vi "forceplate_V1.vi"() -> ()   [LabVIEW 2014]
uses:
  typedef.ctl
  <vilib>/Utility/error.llb/DialogType.ctl
  <vilib>/DAQmx/read.llb/DAQmx Read (Analog 1D DBL NChan 1Samp).vi
  <vilib>/DAQmx/create/channels.llb/DAQmx Create Channel (AI-Voltage-Basic).vi
  <vilib>/DAQmx/miscellaneous.llb/DAQmx Fill In Error Info.vi
  <vilib>/Utility/file.llb/Write To Spreadsheet File (DBL).vi
  <vilib>/DAQmx/configure/timing.llb/DAQmx Timing (Sample Clock).vi
panel:
  in  "save":bool
  out "Kilogram (kg)":dbl
  out "Peak force (N) landing phase":dbl
  out "Peak force (N) contact phase":dbl
  out "Flight time (s)":dbl
  out "Jump height (m)":dbl
  in  "Jump#":dbl=1.0
  out "sampling rate for last data":dbl=1000.0
  out "average":dbl
  out "Slide":dbl(slide) scale=0.0..3000.0
  in  "start":bool
  in  "calibrate":bool
  out "scale":dbl
  out "known":dbl
  out "zero":dbl
  in  "Calibration\n weight (kg)":dbl
  out "Newton (N)":dbl
  in  "Stop":bool
  out "Waveform Graph":dbl[](graph)
  in  "Sample rate":dbl=1000.0
  in  "Sample Clock Source":tag="OnboardClock"
  in  "Terminal Configuration":i32(ring)=-1 items=["default"=-1, "RSE"=10083, "NRSE"=10078, "Differential"=10106, "Pseudodifferential"=12529]
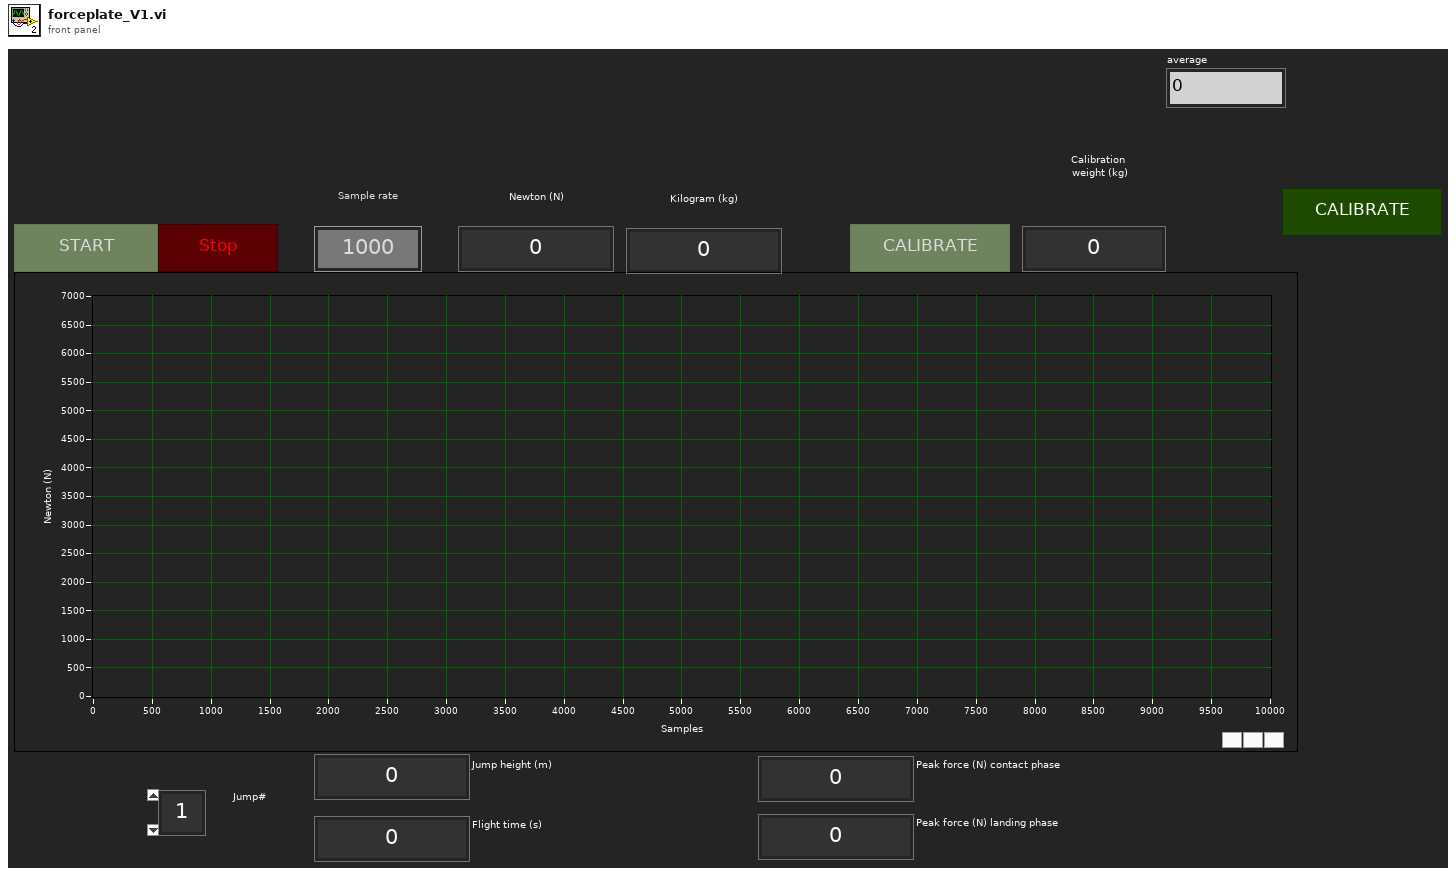
[diagram p1: front panel]
types:
  T1 = typedef "typedef.ctl" = enum16{"display", "read", "calibrate", "wait", "Init"}
  T2 = enum8{"Enabled", "Disabled", "Disabled and Grayed Out"}
  T3 = typedef "DialogType.ctl" = u16
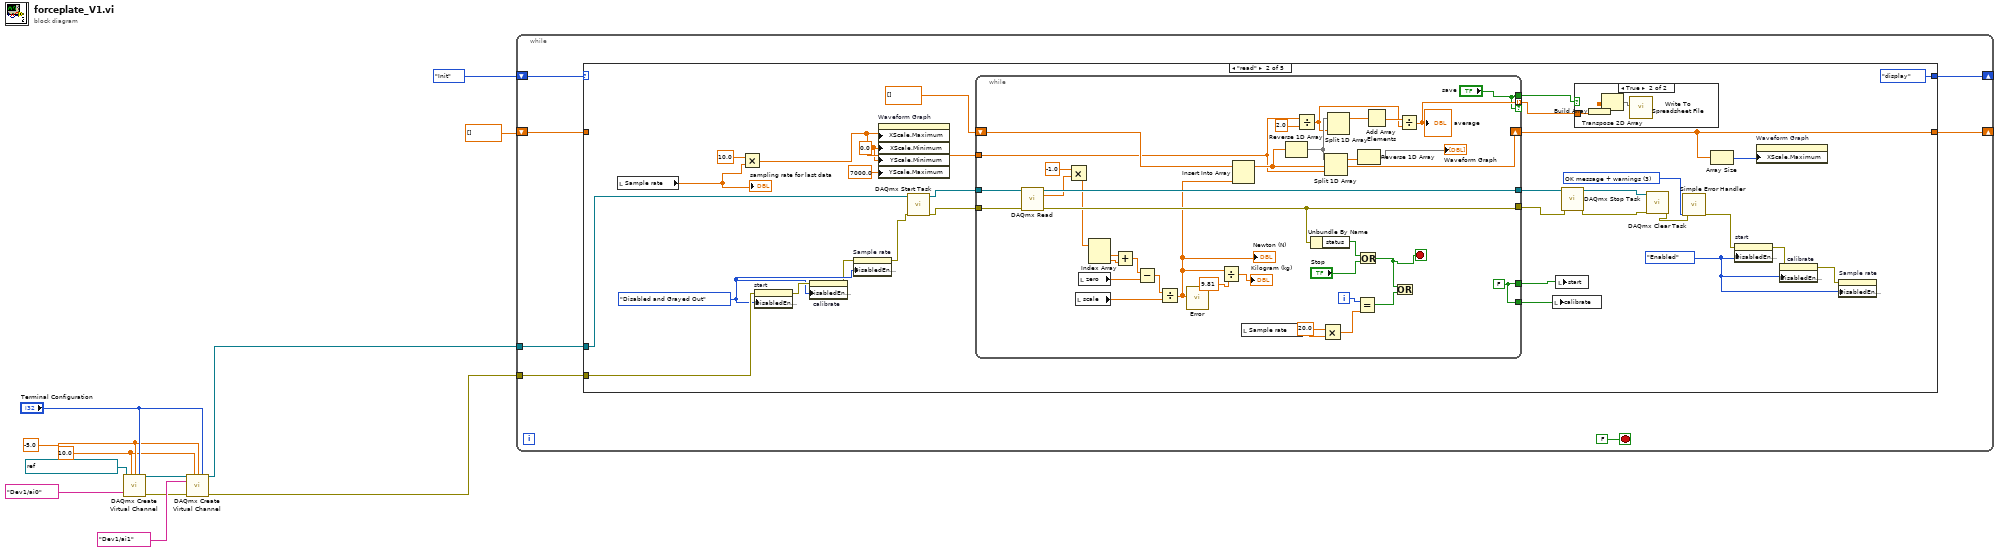
[diagram p0: block diagram]
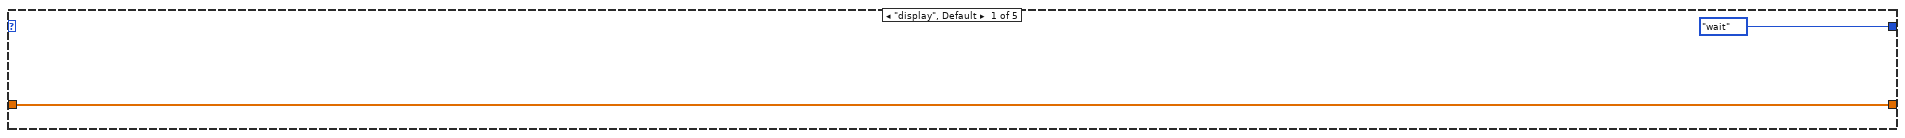
[diagram p2: hidden frame]
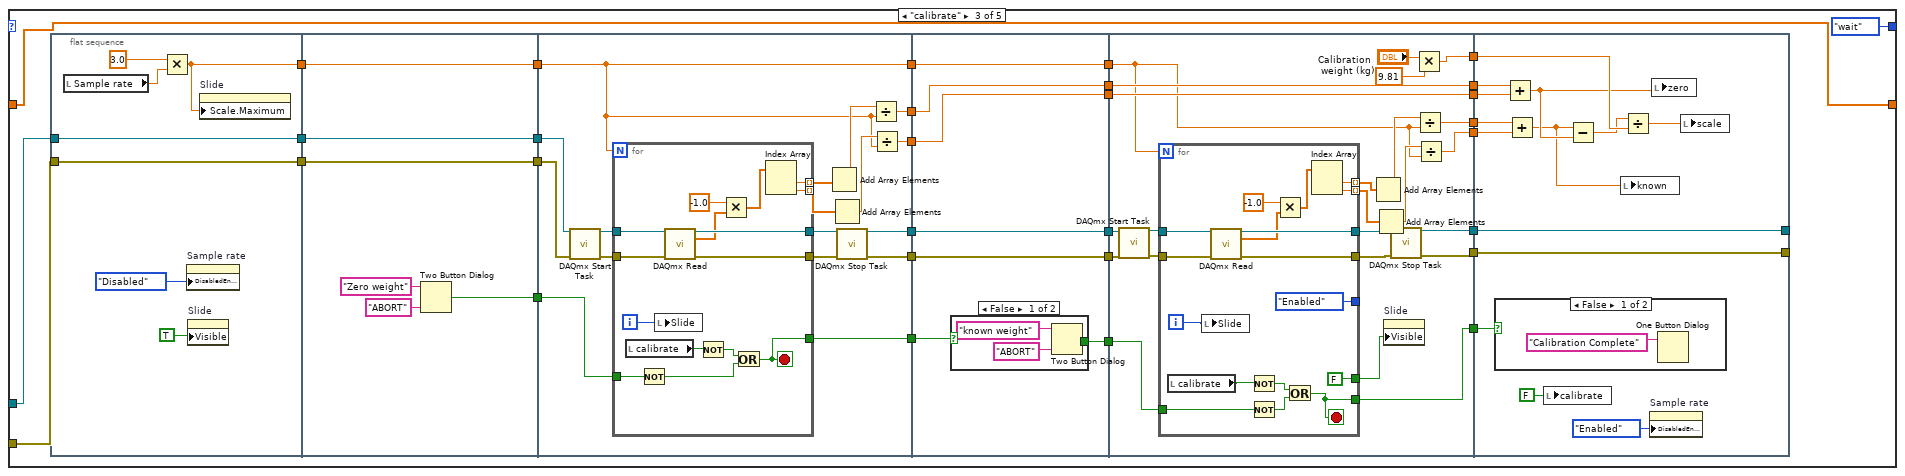
[diagram p4: hidden frame]
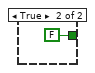
[diagram p5: hidden frame]
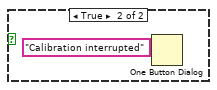
[diagram p6: hidden frame]
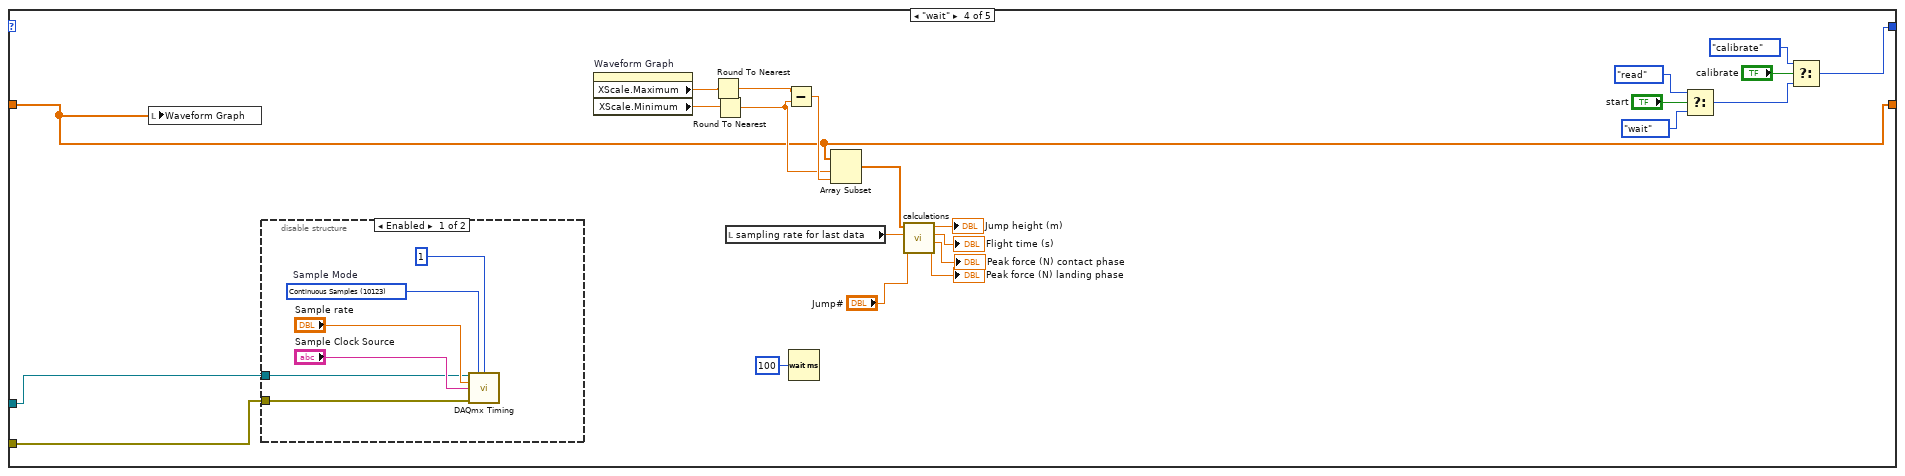
[diagram p7: hidden frame]
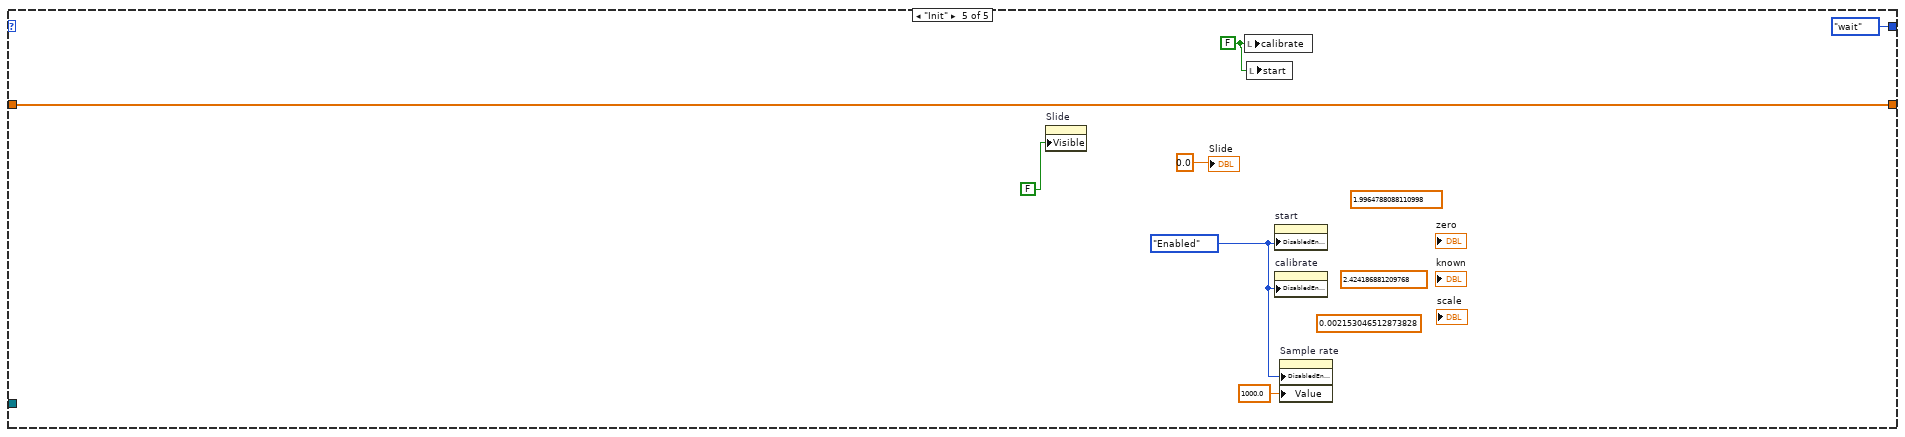
[diagram p9: hidden frame]
diagram:
  w6 = -5.0 ("Min Voltage")
  w5 = 10.0 ("Max Voltage")
  n1 = call-poly <vilib>:"DAQmx Create Virtual Channel.vi"("task in"=refnum<k21> "ProjectVoltageTask", "maximum value"=w5, "minimum value"=w6, "input terminal configuration"="Terminal Configuration", "physical channels"=tag "Dev1/ai0" ("Physical Channel")) -> ("task out"=w9:refnum<k21>, "error out"=w8:errorcluster)  [unwired: 9 in]
  n2 = call-poly <vilib>:"DAQmx Create Virtual Channel.vi"("task in"=w9, "maximum value"=w5, "minimum value"=w6, "input terminal configuration"="Terminal Configuration", "physical channels"=tag "Dev1/ai1" ("Physical Channel 2"), "error in"=w8) -> ("task out"=w2:refnum<k21>, "error out"=w1:errorcluster)  [unwired: 8 in]
  n3 = while {
    shift-right: [w18] -> _
    shift-left: typedef."Init" ("Enum") -> [w19]
    tunnel: w2 -> [w17]
    tunnel: w1 -> [w16]
    shift-right: [w15] -> _
    shift-left: dbl[] [] -> [w14]
    stop <- FALSE stop-if-true
    n4 = case shown="\"read\"" w19 {
      tunnel: [typedef."wait" ("Enum") typedef."display" ("Enum") typedef."wait" ("Enum") w253 typedef."wait" ("Enum")] -> w18
      tunnel: w17 -> [_ w43 w100 w251 _]
      tunnel: w16 -> [_ w37 w99 w250 _]
      tunnel: [w20 w24 w97 w243 w270] -> w15
      tunnel: w14 -> [w20 _ w97 w243 w270]
      frame "display", Default {
      }
      frame "read" {
        w28 = T2."Enabled" ("Disabled")
        w32 = T2."Disabled and Grayed Out" ("Disabled")
        w27 = 0.0 ("Y Scale.Range:Minimum")
        w49 = T3 3 items=["no dialog", "OK message", "continue or stop message", "OK message + warnings", "continue/stop + warnings"] ("type of dialog (OK msg:1)")
        n5 = local read "Sample rate"() -> (w33:dbl)
        "sampling rate for last data" <- w33
        n6 = Multiply(x=10.0, y=w33) -> (x*y=w40:dbl)
        n7 = property on="start" class="Bool (strict)"(error in=w37, "DisabledEnum"=w32) -> (error out=w35:errorcluster)  [unwired: 1 in, 1 out]
        n8 = property on="calibrate" class="Bool (strict)"(error in=w35, "DisabledEnum"=w32) -> (error out=w30:errorcluster)  [unwired: 1 in, 1 out]
        n9 = property on="Sample rate" class="DigNum (strict)"(error in=w30, "DisabledEnum"=w32) -> (error out=w31:errorcluster)  [unwired: 1 in, 1 out]
        n10 = property on="Waveform Graph" class="WFGraph (strict)"("XScale.Maximum"=w40, "XScale.Minimum"=w27, "YScale.Minimum"=w27, "YScale.Maximum"=7000.0 ("Y Scale.Range:Maximum")) -> ()  [unwired: 2 in, 2 out]
        n11 = call <vilib>:"DAQmx Start Task.vi"("task/channels in"=w43, "error in"=w31) -> ("task out"=w51:refnum<k21>, "error out"=w52:errorcluster)  [unwired: 12 in]
        n12 = while {
          tunnel: w51 -> [w92]
          tunnel: w52 -> [w91]
          tunnel: [w90] -> w45
          tunnel: [w88] -> w46
          shift-right: [w72] -> w24
          shift-left: dbl[] [] -> [w86]
          tunnel: w40 -> [w65]
          tunnel: [w67] -> w39
          tunnel: [w67] -> w38
          tunnel: [w57] -> w22 mode=indexing if="save"
          tunnel: ["save"] -> w23
          i -> [w76]
          stop <- w68 stop-if-true
          w67 = FALSE ("start")
          n13 = call-poly <vilib>:"DAQmx Read.vi"("task/channels in"=w92, "error in"=w91) -> ("task out"=w90:refnum<k21>, "data"=w83:dbl[], "error out"=w88:errorcluster)  [unwired: 11 in]
          n14 = Multiply(x=-1.0, y=w83) -> (x*y=w82:dbl[])
          n15 = local read "scale"() -> (w79:dbl)
          n16 = local read "zero"() -> (w81:dbl)
          n17 = Index Array(array=w82) -> (element #1=w77:dbl, element #2=w78:dbl)  [unwired: 2 in]
          n18 = Add(x=w77, y=w78) -> (x+y=w69:dbl)
          n19 = Subtract(x=w69, y=w81) -> (x-y=w80:dbl)
          n20 = Divide(x=w80, y=w79) -> (x/y=w58:dbl)
          "Newton (N)" <- w58
          n21 = call "Error.vi"("Newton (N)"=w58) -> ()  [unwired: 10 in, 1 out]
          n22 = Divide(x=w58, y=9.81) -> (x/y=→"Kilogram (kg)":dbl)
          n23 = Insert Into Array(array=w86, new element=w58) -> (w72:dbl[])  [unwired: 1 in]
          n24 = local read "Sample rate"() -> (w75:dbl)
          n25 = Reverse 1D Array(array=w72) -> (reversed array=w66:dbl[])
          n26 = Divide(x=w65, y=2.0) -> (x/y=w61:dbl)
          n27 = Unbundle By Name(w88) -> ("status"=w87:bool)
          n28 = Multiply(x=20.0, y=w75) -> (x*y=w73:dbl)
          n29 = Split 1D Array(array=w66, index=w65) -> (first subarray=w85:dbl[])  [unwired: 1 out]
          n30 = Split 1D Array(array=w66, index=w61) -> (first subarray=w63:dbl[])  [unwired: 1 out]
          n31 = Equal?(x=w76, y=w73) -> (x = y?=w70:bool)
          n32 = Or(x=w87, y="Stop") -> (x .or. y?=w68:bool)
          n33 = Reverse 1D Array(array=w85) -> (reversed array=→"Waveform Graph":dbl[])
          n34 = Add Array Elements(numeric array=w63) -> (sum=w62:dbl)
          n35 = Or(x=w68, y=w70) -> ()  [unwired: 1 out]
          n36 = Divide(x=w62, y=w61) -> (x/y=w57:dbl)
          "average" <- w57
        }
        n37 = local write "calibrate"(w38) -> ()
        n38 = local write "start"(w39) -> ()
        n39 = call <vilib>:"DAQmx Stop Task.vi"("task/channels in"=w45, "error in"=w46) -> ("task out"=w48:refnum<k21>, "error out"=w47:errorcluster)  [unwired: 12 in]
        n40 = case shown="True" w23 {
          tunnel: w22 -> [_ w55]
          frame False {
          }
          frame True {
            n41 = Build Array(w55) -> (w54:dbl[][])
            n42 = Transpose 2D Array(2D array=w54) -> (transposed array=w53:dbl[][])
            n43 = call-poly <vilib>:"Write To Spreadsheet File.vi"("2D data"=w53) -> ()  [unwired: 7 in, 1 out]
          }
        }
        n44 = call <vilib>:"DAQmx Clear Task.vi"("task in"=w48, "error in"=w47) -> ("error out"=w44:errorcluster)  [unwired: 13 in]
        n45 = call <vilib>:"Simple Error Handler.vi"("type of dialog (OK msg:1)"=w49, "error in (no error)"=w44) -> ("error out"=w36:errorcluster)  [unwired: 3 in, 4 out]
        n46 = Array Size(array=w24) -> (size(s)=w25:i32)
        n47 = property on="start" class="Bool (strict)"(error in=w36, "DisabledEnum"=w28) -> (error out=w34:errorcluster)  [unwired: 1 in, 1 out]
        n48 = property on="Waveform Graph" class="WFGraph (strict)"("XScale.Maximum"=w25) -> ()  [unwired: 2 in, 2 out]
        n49 = property on="calibrate" class="Bool (strict)"(error in=w34, "DisabledEnum"=w28) -> (error out=w29:errorcluster)  [unwired: 1 in, 1 out]
        n50 = property on="Sample rate" class="DigNum (strict)"(error in=w29, "DisabledEnum"=w28) -> ()  [unwired: 1 in, 2 out]
      }
      frame "calibrate" {
        n51 = flat-sequence {
          tunnel: w99 -> [w129]
          tunnel: w100 -> [w130]
          tunnel: [w130] -> w123
          tunnel: [w129] -> w122
          tunnel: [w124] -> w121
          tunnel: [w136] -> w120
          tunnel: [w135] -> w119
          tunnel: w123 -> [w136]
          tunnel: w122 -> [w135]
          tunnel: [w131] -> w118
          tunnel: w121 -> [w131]
          tunnel: [w132] -> w95
          tunnel: w120 -> [w141]
          tunnel: w119 -> [w140]
          tunnel: [w149] -> w117
          tunnel: [w148] -> w116
          tunnel: [w146] -> w115
          tunnel: [w144] -> w114
          tunnel: [w139] -> w113
          tunnel: w118 -> [w139]
          tunnel: w95 -> [w138]
          tunnel: [w137] -> w94
          tunnel: w117 -> [w172]
          tunnel: w116 -> [w171]
          tunnel: [w175] -> w112
          tunnel: w115 -> [w175]
          tunnel: [w174] -> w111
          tunnel: w114 -> [w174]
          tunnel: [w173] -> w110
          tunnel: w113 -> [w173]
          tunnel: [w172] -> w109
          tunnel: [w171] -> w108
          tunnel: w94 -> [w170]
          tunnel: [w169] -> w93
          tunnel: w112 -> [w194]
          tunnel: w111 -> [w192]
          tunnel: w110 -> [w183]
          tunnel: w109 -> [w196]
          tunnel: w108 -> [w195]
          tunnel: [w198] -> w107
          tunnel: [w197] -> w106
          tunnel: [w185] -> w105
          tunnel: [w196] -> w104
          tunnel: [w195] -> w103
          tunnel: [w188] -> w102
          tunnel: [w187] -> w101
          tunnel: [w182] -> w96
          tunnel: w93 -> [w180]
          tunnel: w107 -> [w229]
          tunnel: w106 -> [w228]
          tunnel: w105 -> [w233]
          tunnel: w104 -> [w231]
          tunnel: w103 -> [w230]
          tunnel: w102 -> [w223]
          tunnel: w101 -> [w232]
          tunnel: [w223] -> _
          tunnel: [w232] -> _
          tunnel: w96 -> [w220]
          frame #0 {
            n52 = local read "Sample rate"() -> (w127:dbl)
            n53 = Multiply(x=3.0, y=w127) -> (x*y=w124:dbl)
            n54 = property on="Sample rate" class="DigNum (strict)"("DisabledEnum"=T2."Disabled" ("Disabled")) -> ()  [unwired: 2 in, 2 out]
            n55 = property on="Slide" class="Slide (strict)"("Visible"=TRUE) -> ()  [unwired: 2 in, 2 out]
            n56 = property on="Slide" class="Slide (strict)"("Scale.Maximum"=w124) -> ()  [unwired: 2 in, 2 out]
          }
          frame #1 {
            n57 = Two Button Dialog(message="Zero weight", 1:"ABORT" ("F button name (\"Cancel\")")) -> (T button?=w132:bool)  [unwired: 1 in]
          }
          frame #2 {
            n58 = call <vilib>:"DAQmx Start Task.vi"("task/channels in"=w141, "error in"=w140) -> ("task out"=w142:refnum<k21>, "error out"=w143:errorcluster)  [unwired: 12 in]
            n59 = for {
              N: w139 -> [_]
              tunnel: w142 -> [w167]
              tunnel: w143 -> [w166]
              tunnel: [w162] -> w153 mode=indexing
              tunnel: [w165] -> w152 mode=indexing
              tunnel: [w164] -> w147
              tunnel: [w163] -> w145
              tunnel: w138 -> [w158]
              tunnel: [w156] -> w137
              i -> [w159]
              stop <- w156 stop-if-true
              n60 = local read "calibrate"() -> (w157:bool)
              n61 = Not(x=w158) -> (.not. x?=w155:bool)
              n62 = local write "Slide"(w159) -> ()
              n63 = call-poly <vilib>:"DAQmx Read.vi"("task/channels in"=w167, "error in"=w166) -> ("task out"=w164:refnum<k21>, "data"=w161:dbl[], "error out"=w163:errorcluster)  [unwired: 11 in]
              n64 = Not(x=w157) -> (.not. x?=w154:bool)
              n65 = Multiply(x=-1.0, y=w161) -> (x*y=w160:dbl[])
              n66 = Or(x=w154, y=w155) -> (x .or. y?=w156:bool)
              n67 = Index Array(array=w160) -> (element #1=w162:dbl, element #2=w165:dbl)  [unwired: 2 in]
            }
            n68 = Add Array Elements(numeric array=w153) -> (sum=w151:dbl)
            n69 = Add Array Elements(numeric array=w152) -> (sum=w150:dbl)
            n70 = call <vilib>:"DAQmx Stop Task.vi"("task/channels in"=w147, "error in"=w145) -> ("task out"=w146:refnum<k21>, "error out"=w144:errorcluster)  [unwired: 12 in]
            n71 = Divide(x=w151, y=w139) -> (x/y=w149:dbl)
            n72 = Divide(x=w150, y=w139) -> (x/y=w148:dbl)
          }
          frame #3 {
            n73 = case shown="False" w170 {
              tunnel: [w176 FALSE ("T button?")] -> w169
              frame False {
                n74 = Two Button Dialog(message="known weight", 1:"ABORT" ("F button name (\"Cancel\")")) -> (T button?=w176:bool)  [unwired: 1 in]
              }
              frame True {
              }
            }
          }
          frame #4 {
            n75 = call <vilib>:"DAQmx Start Task.vi"("task/channels in"=w194, "error in"=w192) -> ("task out"=w193:refnum<k21>, "error out"=w191:errorcluster)  [unwired: 12 in]
            n76 = for {
              N: w183 -> [_]
              tunnel: w193 -> [w218]
              tunnel: w191 -> [w217]
              tunnel: [w216] -> w200 mode=indexing
              tunnel: [w215] -> w199 mode=indexing
              tunnel: [T2."Enabled" ("Disabled")] -> _
              tunnel: [w213] -> w190
              tunnel: [w212] -> w189
              tunnel: [w203] -> w182
              tunnel: [FALSE ("Visible")] -> w181
              tunnel: w180 -> [w204]
              i -> [w209]
              stop <- w203 stop-if-true
              n77 = local read "calibrate"() -> (w207:bool)
              n78 = local write "Slide"(w209) -> ()
              n79 = call-poly <vilib>:"DAQmx Read.vi"("task/channels in"=w218, "error in"=w217) -> ("task out"=w213:refnum<k21>, "data"=w211:dbl[], "error out"=w212:errorcluster)  [unwired: 11 in]
              n80 = Not(x=w207) -> (.not. x?=w205:bool)
              n81 = Not(x=w204) -> (.not. x?=w206:bool)
              n82 = Multiply(x=-1.0, y=w211) -> (x*y=w210:dbl[])
              n83 = Or(x=w205, y=w206) -> (x .or. y?=w203:bool)
              n84 = Index Array(array=w210) -> (element #1=w216:dbl, element #2=w215:dbl)  [unwired: 2 in]
            }
            n85 = Add Array Elements(numeric array=w200) -> (sum=w201:dbl)
            n86 = Add Array Elements(numeric array=w199) -> (sum=w202:dbl)
            n87 = property on="Slide" class="Slide (strict)"("Visible"=w181) -> ()  [unwired: 2 in, 2 out]
            n88 = call <vilib>:"DAQmx Stop Task.vi"("task/channels in"=w190, "error in"=w189) -> ("task out"=w188:refnum<k21>, "error out"=w187:errorcluster)  [unwired: 12 in]
            n89 = Multiply(x="Calibration\n weight (kg)", y=9.81) -> (x*y=w185:dbl)
            n90 = Divide(x=w201, y=w183) -> (x/y=w198:dbl)
            n91 = Divide(x=w202, y=w183) -> (x/y=w197:dbl)
          }
          frame #5 {
            n92 = case shown="False" w220 {
              frame False {
                n93 = One Button Dialog(message="Calibration Complete") -> ()  [unwired: 1 in, 1 out]
              }
              frame True {
                n94 = One Button Dialog(message="Calibration interrupted") -> ()  [unwired: 1 in, 1 out]
              }
            }
            n95 = Add(x=w231, y=w230) -> (x+y=w227:dbl)
            n96 = Add(x=w229, y=w228) -> (x+y=w225:dbl)
            n97 = local write "calibrate"(FALSE ("calibrate")) -> ()
            n98 = Subtract(x=w225, y=w227) -> (x-y=w226:dbl)
            n99 = local write "known"(w225) -> ()
            n100 = Divide(x=w226, y=w233) -> (x/y=w224:dbl)
            n101 = property on="Sample rate" class="DigNum (strict)"("DisabledEnum"=T2."Enabled" ("Disabled")) -> ()  [unwired: 2 in, 2 out]
            n102 = local write "zero"(w227) -> ()
            n103 = local write "scale"(w224) -> ()
          }
        }
      }
      frame "wait" {
        n104 = local write "Waveform Graph"(w243) -> ()
        n105 = disable-structure shown="Enabled" {
          disable-tunnel: w251 -> [w260 _]
          disable-tunnel: w250 -> [w259 _]
          frame Enabled {
            w262 = 10123 items=["Finite Samples"=10178, "Continuous Samples"=10123, "Hardware Timed Single Point"=12522]  # Sample Mode
            n106 = call-poly <vilib>:"DAQmx Timing.vi"("task/channels in"=w260, "sample mode"=w262, "samples per channel"=1 ("Number of Samples"), "rate"="Sample rate", "source"="Sample Clock Source", "error in"=w259) -> ()  [unwired: 8 in, 2 out]
          }
          frame Disabled {
          }
        }
        n107 = property on="Waveform Graph" class="WFGraph (strict)"() -> ("XScale.Maximum"=w249:dbl, "XScale.Minimum"=w248:dbl)  [unwired: 2 in, 2 out]
        n108 = Round To Nearest(number=w249) -> (nearest integer value=w247:dbl)
        n109 = Round To Nearest(number=w248) -> (nearest integer value=w245:dbl)
        n110 = local read "sampling rate for last data"() -> (w244:dbl)
        n111 = Subtract(x=w247, y=w245) -> (x-y=w246:dbl)
        n112 = Wait (ms)(milliseconds to wait=u32 100) -> ()  [unwired: 1 out]
        n113 = Array Subset(array=w243, index=w245, length=w246) -> (w242:dbl[])
        n114 = call "calculations.vi"("Jump"="Jump#", "Sampling rate"=w244, "Force data"=w242) -> ("Peak landing force"=→"Peak force (N) landing phase":dbl, "Peak force"=→"Peak force (N) contact phase":dbl, "flight time"=→"Flight time (s)":dbl, "Jump height"=→"Jump height (m)":dbl)  [unwired: 5 in]
        n115 = Select(t=typedef."read" ("Enum"), s="start", f=typedef."wait" ("Enum")) -> (s? t:f=w254:T1)
        n116 = Select(t=typedef."calibrate" ("Enum"), s="calibrate", f=w254) -> (s? t:f=w253:T1)
      }
      frame "Init" {
        (unwired) 0.002153046512873828 ("scale 2")
        (unwired) 2.424186881209768 ("known 2")
        (unwired) 1.9964788088110998 ("zero 2")
        w268 = T2."Enabled" ("Disabled")
        w269 = FALSE ("calibrate")
        n117 = property on="Slide" class="Slide (strict)"("Visible"=FALSE) -> ()  [unwired: 2 in, 2 out]
        n118 = local write "calibrate"(w269) -> ()
        n119 = local write "start"(w269) -> ()
        n120 = property on="start" class="Bool (strict)"("DisabledEnum"=w268) -> ()  [unwired: 2 in, 2 out]
        n121 = property on="calibrate" class="Bool (strict)"("DisabledEnum"=w268) -> ()  [unwired: 2 in, 2 out]
        n122 = property on="Sample rate" class="DigNum (strict)"("DisabledEnum"=w268, "Value"=1000.0 ("Sample rate")) -> ()  [unwired: 2 in, 2 out]
        "Slide" <- 0.0 ("Slide")
      }
    }
  }
